vi "PlayWithSync_second.vi"() -> ()   [LabVIEW 2017]
uses:
  a2924e48-ab58-445b-922b-c6ebaf42a484.vi
  <vilib>/DAQmx/write.llb/DAQmx Write (Digital Wfm 1Chan NSamp).vi
  <vilib>/Waveform/DWDTOps.llb/DWDT Analog to Digital.vi
  <vilib>/DAQmx/create/channels.llb/DAQmx Create Channel (DO-Digital Output).vi
  <vilib>/DAQmx/configure/trigger.llb/DAQmx Start Trigger (Digital Edge).vi
  <vilib>/DAQmx/configure/timing.llb/DAQmx Timing (Use Waveform).vi
  <vilib>/Waveform/DWDTOps.llb/DWDT Uncompress Digital.vi
  <vilib>/DAQmx/miscellaneous.llb/DAQmx Fill In Error Info.vi
panel:
  in  "Analog Output Start Trigger Source":tag="/Dev1/ao/SampleClock"
  in  "Analog Output Sample Clock Source":tag="/Dev1/ao/SampleClock"
  in  "Line(s)":tag="Dev1/port0/line0"
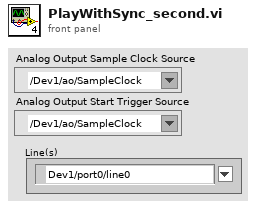
[diagram p1: front panel]
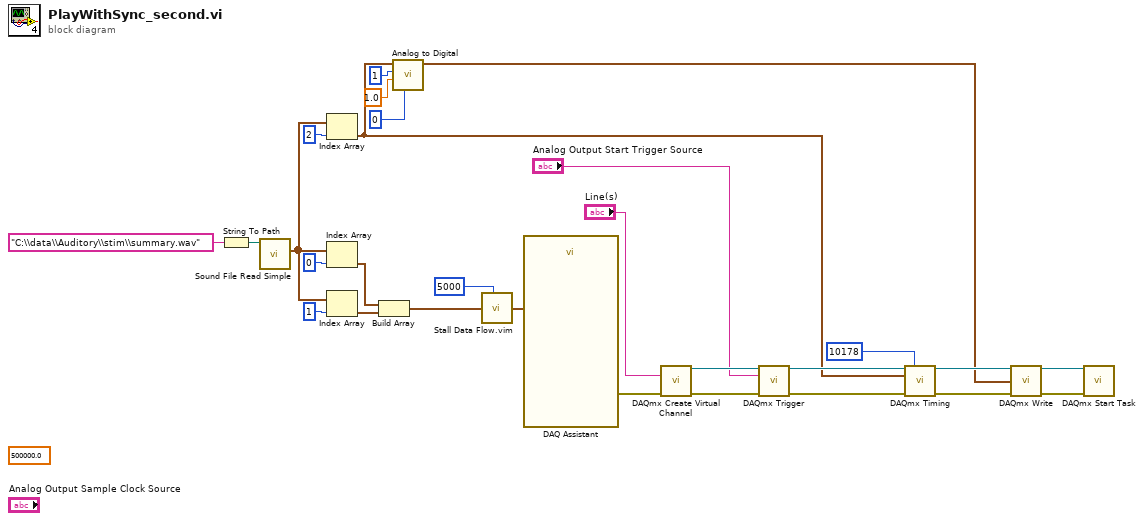
[diagram p0: block diagram]
diagram:
  (unwired) 500000.0
  n1 = String To Path(string="C:\\data\\Auditory\\stim\\summary.wav") -> (path=w28:path)
  n2 = call <vilib>:"Sound File Read Simple.vi"("path"=w28) -> ("data"=w23:waveform(dbl)[])  [unwired: 7 in, 3 out]
  n3 = Index Array(array=w23, index=2) -> (element=w2:waveform(dbl))
  n4 = Index Array(array=w23, index=0) -> (element=w22:waveform(dbl))
  n5 = Index Array(array=w23, index=1) -> (element=w21:waveform(dbl))
  n6 = Build Array(w22, w21) -> (w6:waveform(dbl)[])
  n7 = call-poly <vilib>:"Analog to Digital.vi"("data format (offset binary)"=0, "full-scale range (pk-pk)"=1.0, "resolution (16 bit)"=1, "analog waveform"=w2) -> ("digital waveform"=w3:digitalwaveform)  [unwired: 4 in, 3 out]
  n8 = call "Stall Data Flow.vim"("value in"=w6, "milliseconds to wait"=5000) -> ("value out"=w5:waveform(dbl)[])  [unwired: 1 out]
  n9 = call "DAQ Assistant"("data"=w5) -> ("error out"=w13:errorcluster)  [unwired: 17 in, 1 out]
  n10 = call-poly <vilib>:"DAQmx Create Virtual Channel.vi"("lines"="Line(s)", "error in"=w13) -> ("task out"=w16:refnum<k21>, "error out"=w12:errorcluster)  [unwired: 12 in]
  n11 = call-poly <vilib>:"DAQmx Trigger.vi"("task/channels in"=w16, "source"="Analog Output Start Trigger Source", "error in"=w12) -> ("task out"=w15:refnum<k21>, "error out"=w11:errorcluster)  [unwired: 11 in]
  n12 = call-poly <vilib>:"DAQmx Timing.vi"("task/channels in"=w15, "sample mode"=10178, "waveform"=w2, "error in"=w11) -> ("task out"=w9:refnum<k21>, "error out"=w10:errorcluster)  [unwired: 10 in]
  n13 = call-poly <vilib>:"DAQmx Write.vi"("task/channels in"=w9, "data"=w3, "error in"=w10) -> ("task out"=w8:refnum<k21>, "error out"=w7:errorcluster)  [unwired: 10 in, 1 out]
  n14 = call <vilib>:"DAQmx Start Task.vi"("task/channels in"=w8, "error in"=w7) -> ()  [unwired: 12 in, 2 out]
